vi "quiz3.1.vi"() -> ()   [LabVIEW 2017]
panel:
  out "Tab Control":enum32{"Login", "Menu", "Add", "delete"}(tab)
  in  "Ingresar":bool
  in  "Contraseña":string
  in  "Usuario":string
  in  "Delete Button":bool
  in  "Add Button":bool
  in  "Home Button":bool
  out "Cusuario":string
  in  "Previous Button":bool
  in  "AddContraseña":string
  in  "AddUsuario":string
  in  "Agregar":bool
  out "Agregado":bool
  in  "Cancel Button":bool
  in  "DeleteUsuario 2":string
  in  "Previous Button 2":bool
  out "text":string
  # "USTED INGRESO CON EL USUARIO"
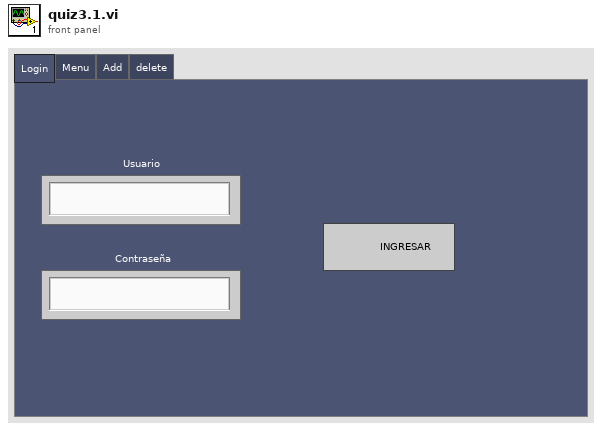
[diagram p1: front panel]
types:
  T1 = enum16{"open", "replace", "create", "open or create", "replace or create", "replace or create with confirmation"}
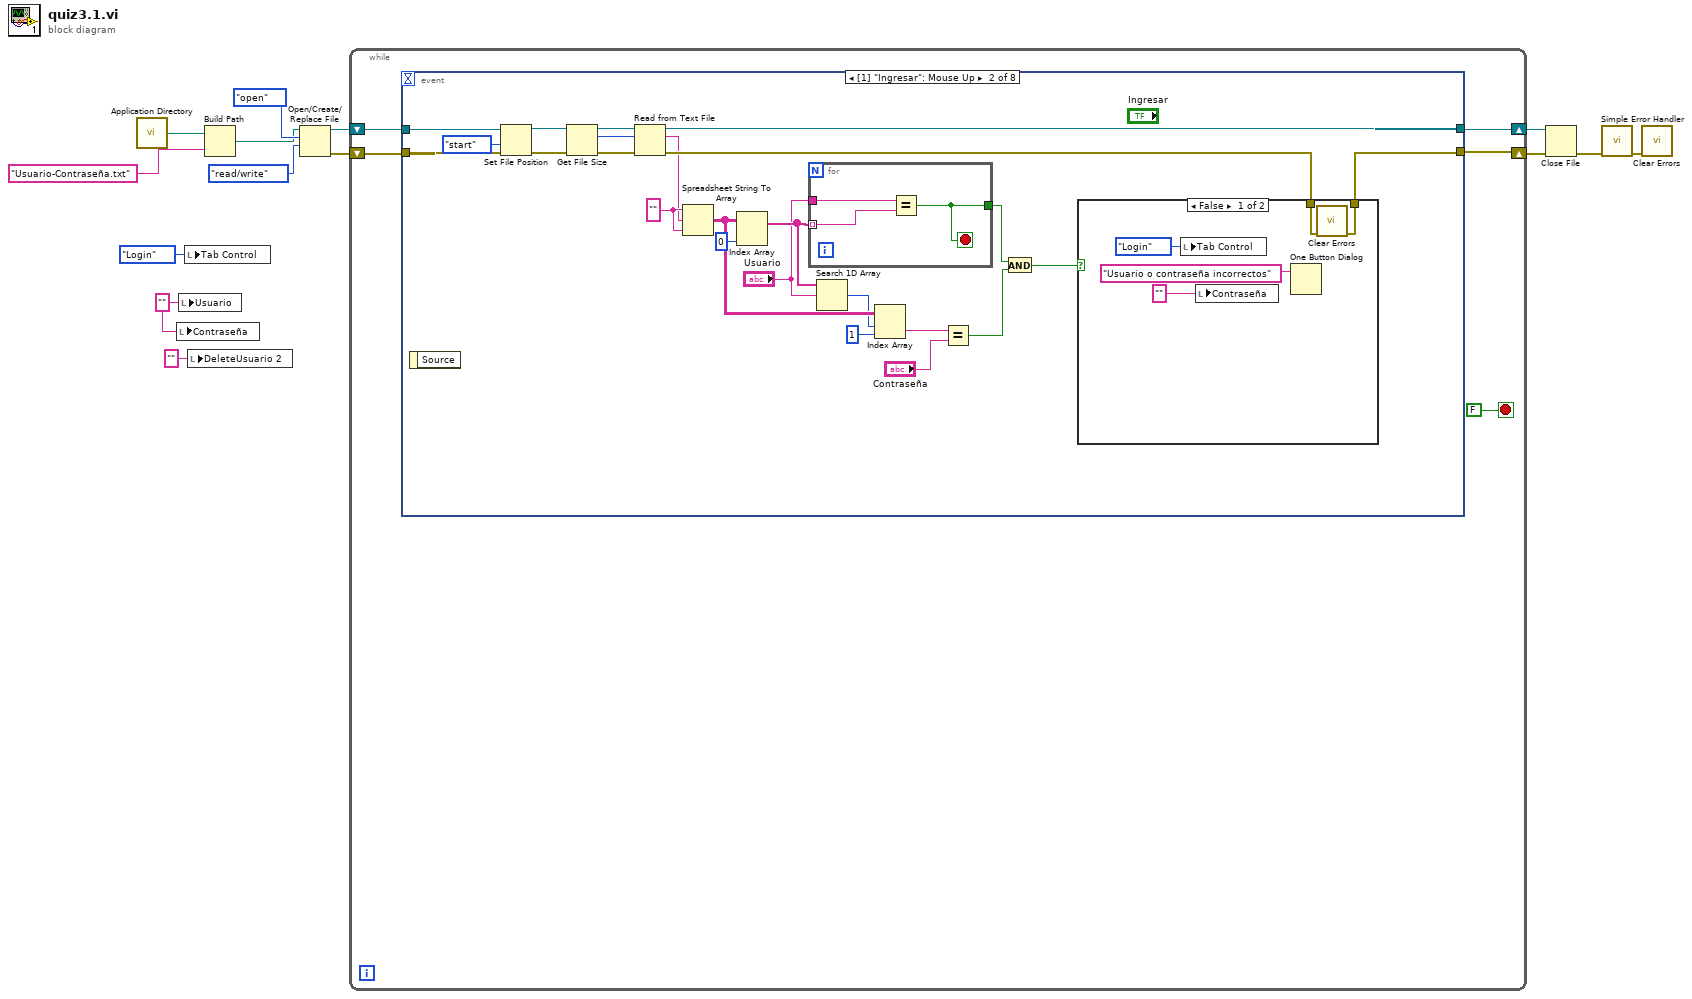
[diagram p0: block diagram]
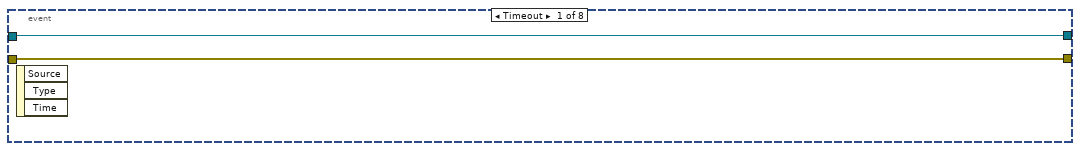
[diagram p2: hidden frame]
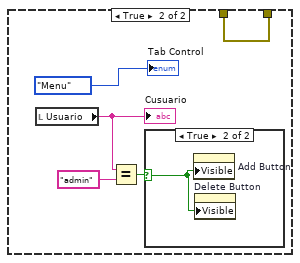
[diagram p3: hidden frame]
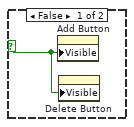
[diagram p4: hidden frame]
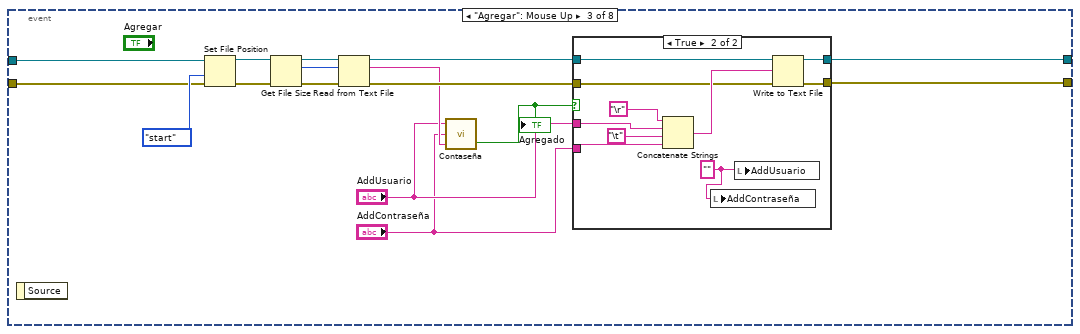
[diagram p5: hidden frame]
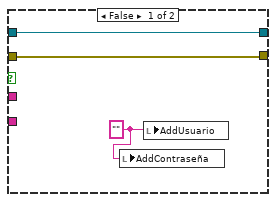
[diagram p6: hidden frame]
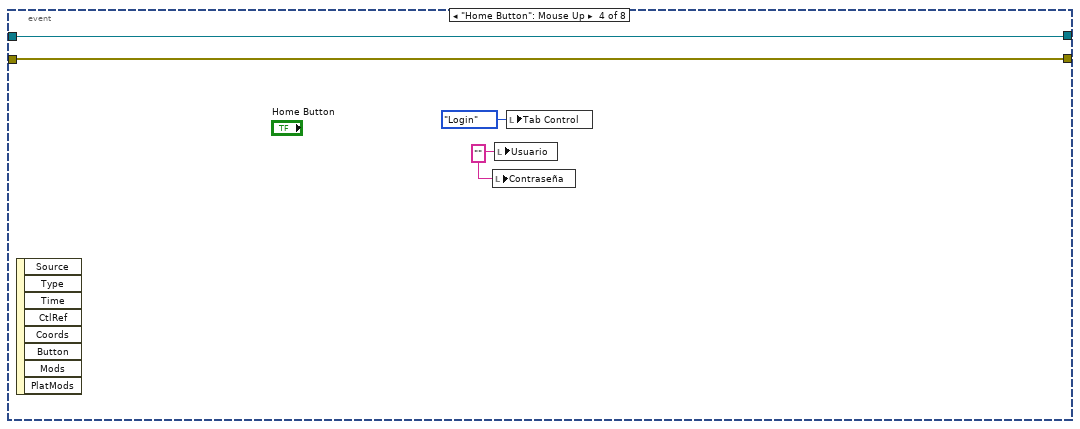
[diagram p7: hidden frame]
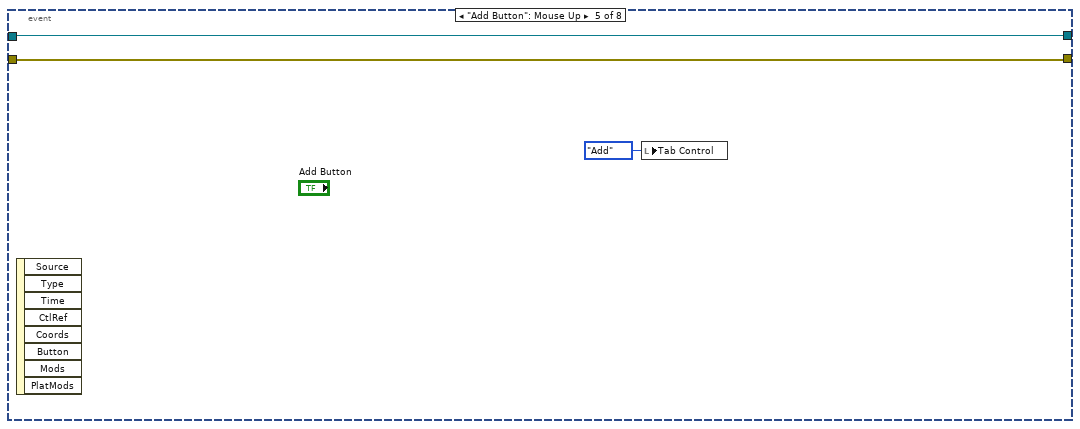
[diagram p8: hidden frame]
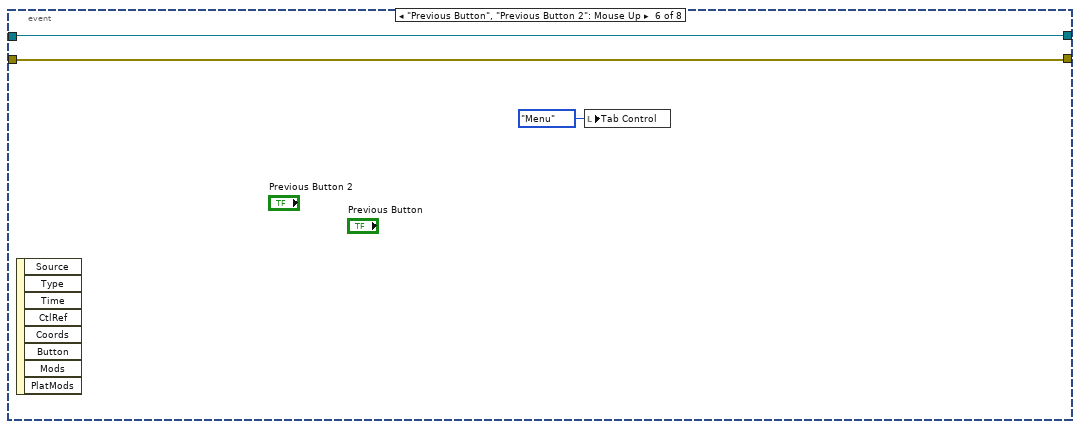
[diagram p9: hidden frame]
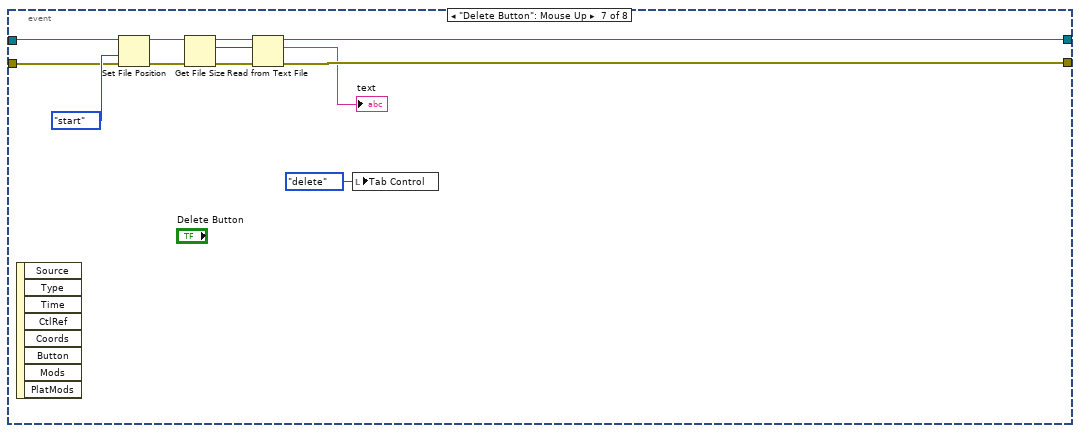
[diagram p10: hidden frame]
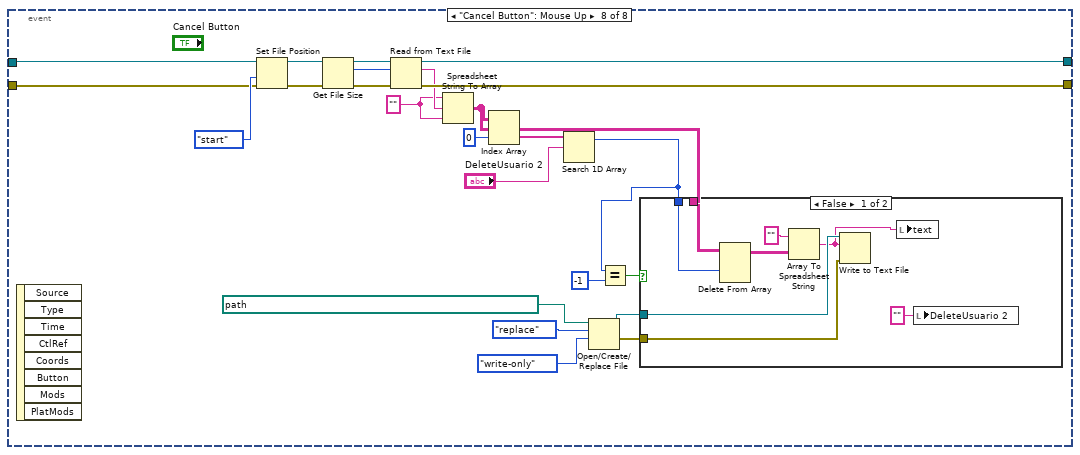
[diagram p11: hidden frame]
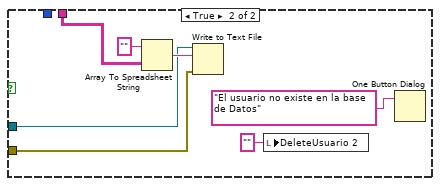
[diagram p12: hidden frame]
diagram:
  w5 = "" ("Usuario")
  n1 = call <vilib>:"Application Directory.vi"() -> ("Application Directory"=w14:path)
  n2 = local write "Contraseña"(w5) -> ()
  n3 = local write "Usuario"(w5) -> ()
  n4 = local write "Tab Control"(enum32{"Login", "Menu", "Add", "delete"}."Login" ("Tab Control")) -> ()
  n5 = local write "DeleteUsuario 2"("" ("DeleteUsuario 2")) -> ()
  n6 = Build Path(base path=w14, name or relative path="Usuario-Contraseña.txt") -> (appended path=w6:path)
  n7 = Open/Create/Replace File(file path (use dialog)=w6, operation (0:open)=T1."open", access (0:read/write)=enum16{"read/write", "read-only", "write-only"}."read/write") -> (refnum out=w2:refnum<file>, error out=w1:errorcluster)  [unwired: 3 in, 1 out]
  n8 = while {
    shift-right: [w16] -> w8
    shift-left: w2 -> [w17]
    shift-right: [w15] -> w7
    shift-left: w1 -> [w18]
    stop <- FALSE stop-if-true
    n9 = event shown="[1] \"Ingresar\": Mouse Up" {
      selector: _ -> [_ _ _ _ _ _ _ _]
      dyn-events: _ -> [_ _ _ _ _ _ _ _]
      timeout: _ -> [_ _ _ _ _ _ _ _]
      tunnel: w18 -> [w20 w45 w64 w91 w95 w98 w102 w129]
      tunnel: [w21 w40 w76 w92 w96 w99 w103 w125] -> w16
      tunnel: [w20 w37 w75 w91 w95 w98 w101 w124] -> w15
      tunnel: w17 -> [w21 w39 w65 w92 w96 w99 w104 w128]
      event Timeout {
        n10 = event-data() -> ()  [unwired: 1 in, 3 out]
      }
      event "Ingresar": Mouse Up {
        w33 = "" ("format string")
        n11 = event-data() -> ()  [unwired: 1 in, 1 out]
        n12 = Set File Position(refnum=w39, from (0:start)=enum16{"start", "end", "current"}."start", error in=w45) -> (refnum out=w43:refnum<file>, error out=w44:errorcluster)  [unwired: 1 in]
        n13 = Get File Size(file=w43, error in=w44) -> (refnum out=w35:refnum<file>, size (in bytes)=w42:i64, 0:w41:errorcluster)
        n14 = Read from Text File(file (use dialog)=w35, count=w42, error in=w41) -> (refnum out=w40:refnum<file>, text=w32:string, error out=w38:errorcluster)  [unwired: 1 in, 1 out]
        n15 = Spreadsheet String To Array(format string=w33, spreadsheet string=w32, array type (2D Dbl)=w33) -> (array=w28:string[][])  [unwired: 1 in]
        n16 = Index Array(array=w28, index (col)=0 ("index")) -> (element=w30:string[])  [unwired: 1 in]
        n17 = for {
          tunnel: "Usuario" -> [w48]
          tunnel: [w47] -> w31
          tunnel: w30 -> [w46] mode=indexing
          stop <- w47 stop-if-true
          n18 = Equal?(x=w48, y=w46) -> (x = y?=w47:bool)
        }
        n19 = Search 1D Array(1D array=w30, element="Usuario") -> (index of element=w23:i32)  [unwired: 1 in]
        n20 = Index Array(array=w28, index (row)=w23, index (col)=1 ("index")) -> (element=w27:string)
        n21 = Equal?(x=w27, y="Contraseña") -> (x = y?=w25:bool)
        n22 = And(x=w31, y=w25) -> (x .and. y?=w34:bool)
        n23 = case shown="False" w34 {
          tunnel: [w51 w58] -> w37
          tunnel: w38 -> [w50 w58]
          frame False {
            n24 = local write "Tab Control"(enum32{"Login", "Menu", "Add", "delete"}."Login" ("Tab Control")) -> ()
            n25 = local write "Contraseña"("" ("Usuario")) -> ()
            n26 = One Button Dialog(message="Usuario o contraseña incorrectos") -> ()  [unwired: 1 in, 1 out]
            n27 = call <vilib>:"Clear Errors.vi"("error in (no error)"=w50) -> ("error out"=w51:errorcluster)  [unwired: 5 in, 1 out]
          }
          frame True {
            n28 = local read "Usuario"() -> (w56:string)
            "Cusuario" <- w56
            n29 = Equal?(x=w56, y="admin") -> (x = y?=w57:bool)
            n30 = case shown="True" w57 {
              selector: w57 -> [w59 w60]
              frame False {
                n31 = property on="Add Button" class="Bool (strict)"("Visible"=w59) -> ()  [unwired: 2 in, 2 out]
                n32 = property on="Delete Button" class="Bool (strict)"("Visible"=w59) -> ()  [unwired: 2 in, 2 out]
              }
              frame True {
                n33 = property on="Add Button" class="Bool (strict)"("Visible"=w60) -> ()  [unwired: 2 in, 2 out]
                n34 = property on="Delete Button" class="Bool (strict)"("Visible"=w60) -> ()  [unwired: 2 in, 2 out]
              }
            }
            "Tab Control" <- enum32{"Login", "Menu", "Add", "delete"}."Menu" ("Tab Control")
          }
        }
      }
      event "Agregar": Mouse Up {
        n35 = event-data() -> ()  [unwired: 1 in, 1 out]
        n36 = Set File Position(refnum=w65, from (0:start)=enum16{"start", "end", "current"}."start", error in=w64) -> (refnum out=w72:refnum<file>, error out=w73:errorcluster)  [unwired: 1 in]
        n37 = Get File Size(file=w72, error in=w73) -> (refnum out=w69:refnum<file>, size (in bytes)=w71:i64, 0:w70:errorcluster)
        n38 = Read from Text File(file (use dialog)=w69, count=w71, error in=w70) -> (refnum out=w67:refnum<file>, text=w63:string, error out=w66:errorcluster)  [unwired: 1 in, 1 out]
        n39 = call "Contaseña.vi"("spreadsheet string"=w63, "AddContraseña"="AddContraseña", "addUsuario"="AddUsuario") -> ("result"=w74:bool)  [unwired: 1 out]
        "Agregado" <- w74
        n40 = case shown="True" w74 {
          tunnel: [w79 w89] -> w76
          tunnel: [w78 w88] -> w75
          tunnel: w67 -> [w79 w84]
          tunnel: w66 -> [w78 w83]
          tunnel: "AddUsuario" -> [_ w82]
          tunnel: "AddContraseña" -> [_ w81]
          frame False {
            w77 = "" ("Usuario")
            n41 = local write "AddContraseña"(w77) -> ()
            n42 = local write "AddUsuario"(w77) -> ()
          }
          frame True {
            w80 = "" ("Usuario")
            n43 = Concatenate Strings("\r", w82, "\t", w81) -> (w87:string)
            n44 = local write "AddContraseña"(w80) -> ()
            n45 = local write "AddUsuario"(w80) -> ()
            n46 = Write to Text File(file (use dialog)=w84, text=w87, error in=w83) -> (refnum out=w89:refnum<file>, error out=w88:errorcluster)  [unwired: 1 in, 1 out]
          }
        }
      }
      event "Home Button": Mouse Up {
        w93 = "" ("Usuario")
        n47 = event-data() -> ()  [unwired: 1 in, 8 out]
        n48 = local write "Contraseña"(w93) -> ()
        n49 = local write "Usuario"(w93) -> ()
        n50 = local write "Tab Control"(enum32{"Login", "Menu", "Add", "delete"}."Login" ("Tab Control")) -> ()
      }
      event "Add Button": Mouse Up {
        n51 = event-data() -> ()  [unwired: 1 in, 8 out]
        n52 = local write "Tab Control"(enum32{"Login", "Menu", "Add", "delete"}."Add" ("Tab Control")) -> ()
      }
      event "Previous Button", "Previous Button 2": Mouse Up {
        n53 = event-data() -> ()  [unwired: 1 in, 8 out]
        n54 = local write "Tab Control"(enum32{"Login", "Menu", "Add", "delete"}."Menu" ("Tab Control")) -> ()
      }
      event "Delete Button": Mouse Up {
        n55 = event-data() -> ()  [unwired: 1 in, 8 out]
        n56 = Set File Position(refnum=w104, from (0:start)=enum16{"start", "end", "current"}."start", error in=w102) -> (refnum out=w109:refnum<file>, error out=w110:errorcluster)  [unwired: 1 in]
        n57 = Get File Size(file=w109, error in=w110) -> (refnum out=w106:refnum<file>, size (in bytes)=w108:i64, 0:w107:errorcluster)
        n58 = Read from Text File(file (use dialog)=w106, count=w108, error in=w107) -> (refnum out=w103:refnum<file>, text=→"text":string, error out=w101:errorcluster)  [unwired: 1 in, 1 out]
        n59 = local write "Tab Control"(enum32{"Login", "Menu", "Add", "delete"}."delete" ("Tab Control")) -> ()
      }
      event "Cancel Button": Mouse Up {
        w121 = "" ("format string")
        n60 = event-data() -> ()  [unwired: 1 in, 8 out]
        n61 = Set File Position(refnum=w128, from (0:start)=enum16{"start", "end", "current"}."start", error in=w129) -> (refnum out=w134:refnum<file>, error out=w135:errorcluster)  [unwired: 1 in]
        n62 = Get File Size(file=w134, error in=w135) -> (refnum out=w131:refnum<file>, size (in bytes)=w133:i64, 0:w132:errorcluster)
        n63 = Read from Text File(file (use dialog)=w131, count=w133, error in=w132) -> (refnum out=w125:refnum<file>, text=w122:string, error out=w124:errorcluster)  [unwired: 1 in, 1 out]
        n64 = Spreadsheet String To Array(format string=w121, spreadsheet string=w122, array type (2D Dbl)=w121) -> (array=w117:string[][])  [unwired: 1 in]
        n65 = Index Array(array=w117, index (col)=0 ("disabled index (col)")) -> (element=w119:string[])  [unwired: 1 in]
        n66 = Search 1D Array(1D array=w119, element="DeleteUsuario 2") -> (index of element=w113:i32)  [unwired: 1 in]
        n67 = Open/Create/Replace File(file path (use dialog)=path "D:/2019-1/Programacion 2/quiz 3/Usuario-Contraseña.txt", operation (0:open)=T1."replace", access (0:read/write)=enum16{"read/write", "read-only", "write-only"}."write-only") -> (refnum out=w116:refnum<file>, error out=w115:errorcluster)  [unwired: 3 in, 1 out]
        n68 = Equal?(x=w113, y=-1) -> (x = y?=w114:bool)
        n69 = case shown="False" w114 {
          tunnel: w117 -> [w143 w146]
          tunnel: w113 -> [w142 _]
          tunnel: w116 -> [w140 w145]
          tunnel: w115 -> [w139 w144]
          frame False {
            n70 = Delete From Array(array=w143, index (row)=w142) -> (array with subset deleted=w141:string[][])  [unwired: 2 in, 1 out]
            n71 = Array To Spreadsheet String(array=w141, 3:"" ("format string")) -> (spreadsheet string=w137:string)  [unwired: 1 in]
            n72 = Write to Text File(file (use dialog)=w140, text=w137, error in=w139) -> ()  [unwired: 1 in, 3 out]
            n73 = local write "text"(w137) -> ()
            n74 = local write "DeleteUsuario 2"("" ("DeleteUsuario 2")) -> ()
          }
          frame True {
            n75 = Array To Spreadsheet String(array=w146, 3:"" ("format string")) -> (spreadsheet string=w148:string)  [unwired: 1 in]
            n76 = Write to Text File(file (use dialog)=w145, text=w148, error in=w144) -> ()  [unwired: 1 in, 3 out]
            n77 = local write "DeleteUsuario 2"("" ("DeleteUsuario 2")) -> ()
            n78 = One Button Dialog(message="El usuario no existe en la base de Datos") -> ()  [unwired: 1 in, 1 out]
          }
        }
      }
    }
  }
  n79 = Close File(refnum=w8, error in=w7) -> (error out=w9:errorcluster)  [unwired: 1 out]
  n80 = call <vilib>:"Simple Error Handler.vi"("error in (no error)"=w9) -> ("error out"=w10:errorcluster)  [unwired: 4 in, 4 out]
  n81 = call <vilib>:"Clear Errors.vi"("error in (no error)"=w10) -> ()  [unwired: 5 in, 2 out]
